vi "PlotRovers.vi"(3 "UDP Robot Inputs & Status":T1(array[cluster])=[{"Left PWM"=1500, "Right PWM"=1500, "Robot Heading"=0, "UDP Transmitting Port"=61541, "UDP Receiving Port"=61540, "Robot Symbol"="R"}, {"Left PWM"=1500, "Right PWM"=1500, "Robot Heading"=0, "UDP Transmitting Port"=61543, "UDP Receiving Port"=61542, "Robot Symbol"="G"}, {"Left PWM"=1500, "Right PWM"=1500, "Robot Heading"=0, "UDP Transmitting Port"=61545, "UDP Receiving Port"=61544, "Robot Symbol"="B"}, {"Left PWM"=1500, "Right PWM"=1500, "Robot Heading"=0, "UDP Transmitting Port"=0, "UDP Receiving Port"=0, "Robot Symbol"="P"}], 4 "Position Array":i32[][](array[numeric])=[[200, 200], [200, 800], [800, 800], [800, 200], [500, 300], [895, 748], [330, 598], [300, 200], [350, 200]], 5 "Picture In":picture) -> (2 "Picture Out":picture)   [LabVIEW 2012]
panel:
  out "Fill Color":u32(colorbox)=16734710
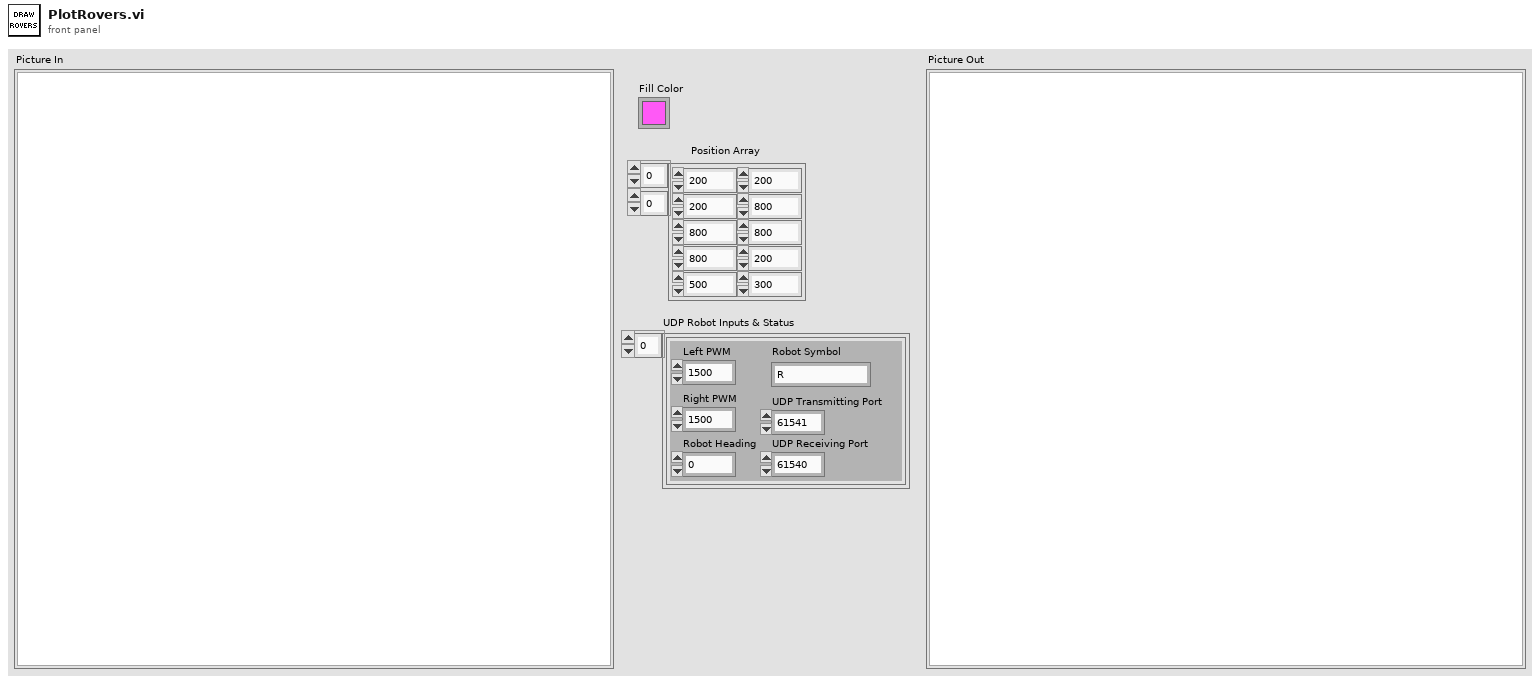
[diagram p1: front panel]
types:
  T1 = cluster{"Left PWM":i32, "Right PWM":i32, "Robot Heading":i32, "UDP Transmitting Port":i32, "UDP Receiving Port":i32, "Robot Symbol":string}[]
  T2 = cluster{"[0]":i16, "[1]":i16, "[2]":i16, "[3]":i16, "[4]":i16, "[5]":i16, "[6]":i16, "[7]":i16, "[8]":i16}
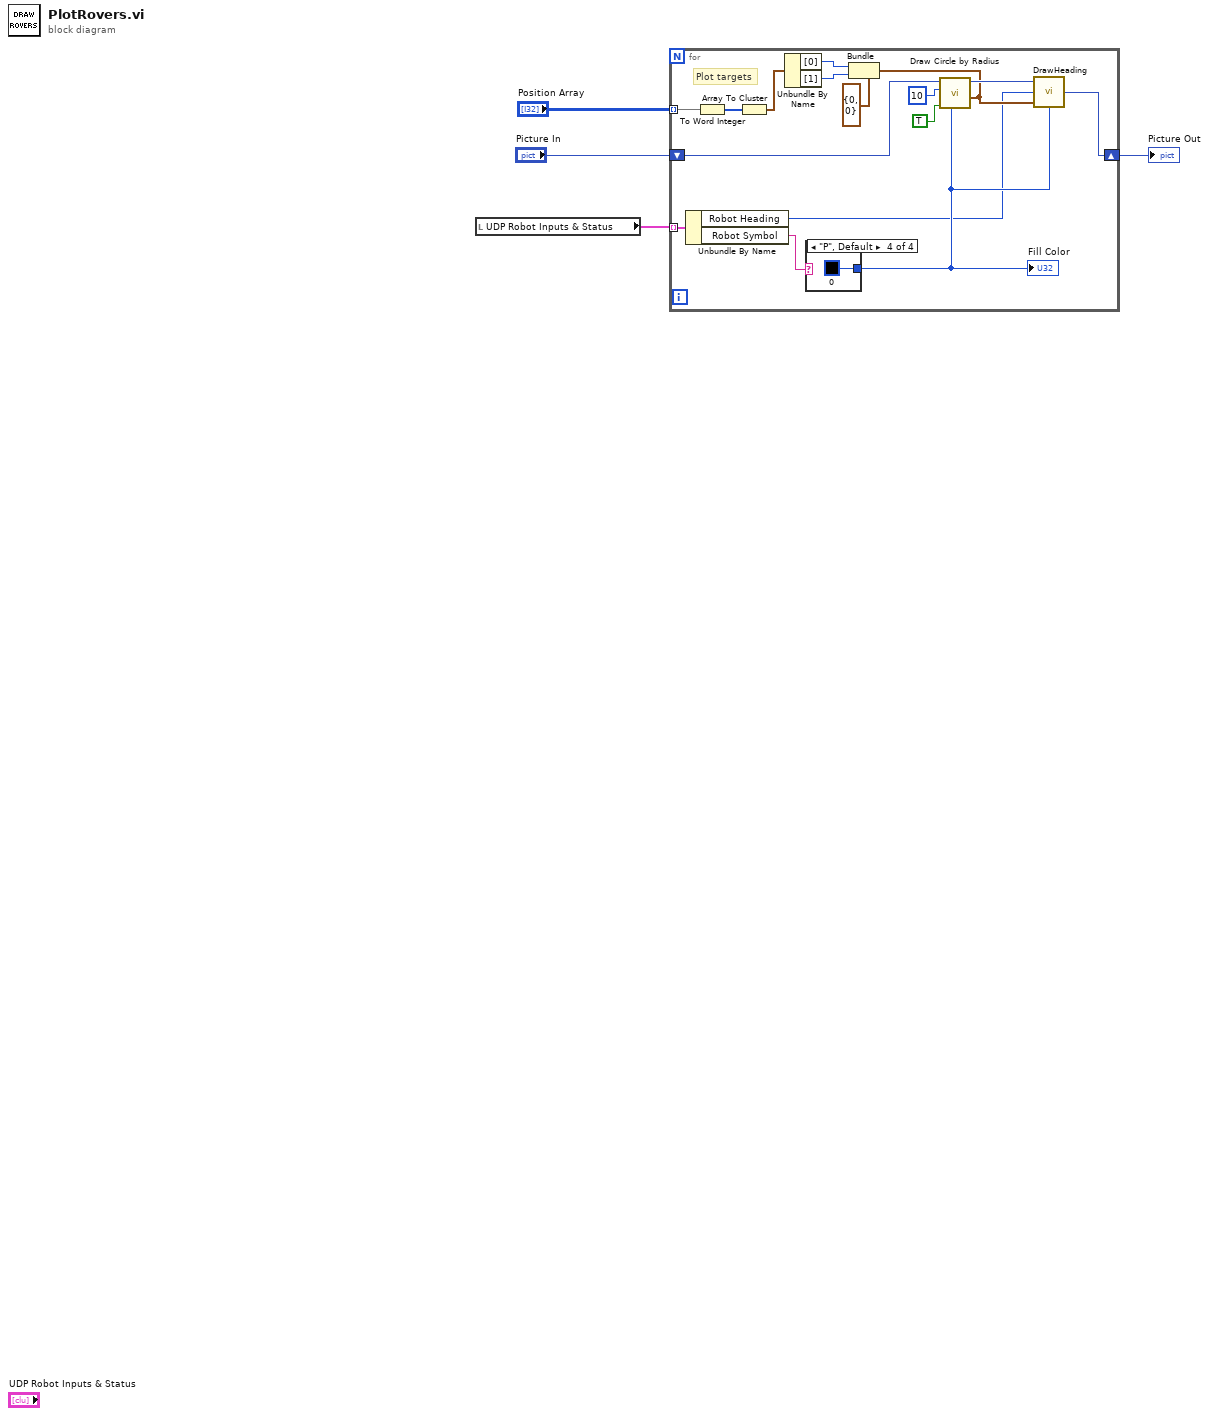
[diagram p0: block diagram]
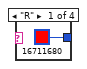
[diagram p2: hidden frame]
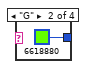
[diagram p3: hidden frame]
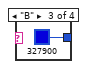
[diagram p4: hidden frame]
diagram:
  n1 = local read "UDP Robot Inputs & Status"() -> (w1:T1)
  n2 = for {
    shift-right: [w9] -> w3
    shift-left: "Picture In" -> [w12]
    tunnel: "Position Array" -> [w18] mode=indexing
    tunnel: w1 -> [w7] mode=indexing
    # "Plot targets"
    n3 = Unbundle By Name(w7) -> ("Robot Heading"=w5:i32, "Robot Symbol"=w6:string)
    n4 = To Word Integer(number=w18) -> (16bit integer=w17:i16[])
    n5 = Array To Cluster(array=w17) -> (cluster=w16:T2)
    n6 = Unbundle By Name(w16) -> ("[0]"=w15:i16, "[1]"=w14:i16)
    n7 = case shown="\"P\", Default" w6 {
      tunnel: [u32 16711680 ("color(black)") u32 6618880 ("color(black)") u32 327900 ("color(black)") u32 0 ("color(black)")] -> w8
      frame "R" {
      }
      frame "G" {
      }
      frame "B" {
      }
      frame "P", Default {
      }
    }
    "Fill Color" <- w8
    n8 = Bundle(cluster=cluster{i16, i16} {0, 0} ("input cluster"), w15, w14) -> (w10:cluster{i16, i16})
    n9 = call <vilib>:"Draw Circle by Radius.vi"("color(black)"=w8, "fill?(F)"=TRUE, "pixel center"=w10, "radius"=i16 10, "picture"=w12) -> ("new picture"=w11:picture)  [unwired: 6 in]
    n10 = call "DrawHeading.vi"("color(black)"=w8, "(xr,yr) old"=w10, "Heading"=w5, "2D Picture"=w11) -> ("new picture"=w9:picture)
  }
  "Picture Out" <- w3
